vi "Polymorphic - Wait.vi"   [LabVIEW 2020]
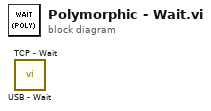
[diagram p0: block diagram]
diagram:
  n1 = call "USB - Wait.vi"() -> ()  [unwired: 10 in, 2 out]
  n2 = call "TCP - Wait.vi"() -> ()  [unwired: 10 in, 2 out]
